vi "ReadCSVTest.vi"() -> (3 "all rows":string[][](array[string]))   [LabVIEW 2019]
uses:
  <vilib>/Utility/file.llb/Read Delimited Spreadsheet (string).vi
panel:
  out "Array":string[](array[string])
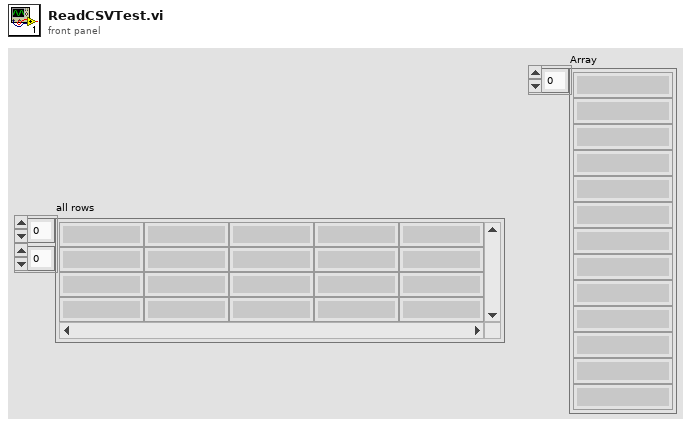
[diagram p1: front panel]
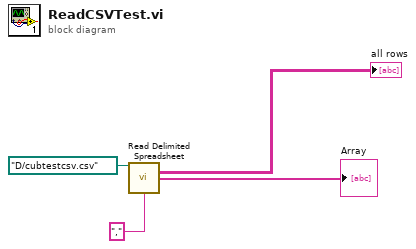
[diagram p0: block diagram]
diagram:
  n1 = call-poly <vilib>:"Read Delimited Spreadsheet.vi"("file path (dialog if empty)"=path "D:/cubtestcsv.csv", "delimiter (\\t)"="," ("delimiter (\\t)")) -> ("all rows"=→"all rows":string[][], "first row"=→"Array":string[])  [unwired: 8 in, 4 out]
